vi "Log In 2.0.vi"(10 "required access level":i32, 11 "Program Root Path":path=path "C:/Labview Code") -> (0 "Password Out":string, 1 "User Name Out":string, 2 "Cancelled":bool, 3 "passed":bool, 4 "Level":i32)   [LabVIEW 2018]
panel:
  in  "User Name":string
  in  "Cancel":bool
  in  "Ok":bool
  in  "Password":string
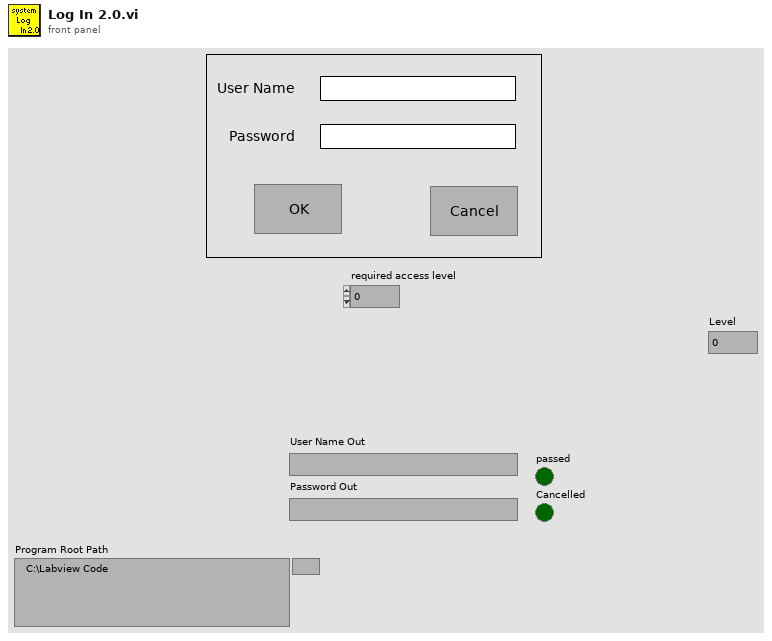
[diagram p1: front panel]
types:
  T1 = cluster{"Program Root Path":path, "Cancelled":bool, "Passed":bool, "User Names":string[], "Passwords":string[], "User Name Index":i32, "access levels":i32[]}
  T2 = typedef "eventvkey.ctl" = enum16{"ASCII", "Enter", "Return", "Shift", "Ctrl", "Alt", "Cmd", "Opt", "Caps", "NumLock", "Clear", "Break", "Up", "Down", "Left", "Right", "Insert", "Delete", "Home", "End", "PageUp", "PageDown", "Escape", "Help", "Pause", "ScrollLock", "F1", "F2", "F3", "F4", "F5", "F6", "F7", "F8", "F9", "F10", "F11", "F12", "F13", "F14", "F15", "F16", "F17", "F18", "F19", "F20", "F21", "F22", "F23", "F24", "Play", "VolumeUp", "VolumeDown", "Mute", "Two Byte Char"}
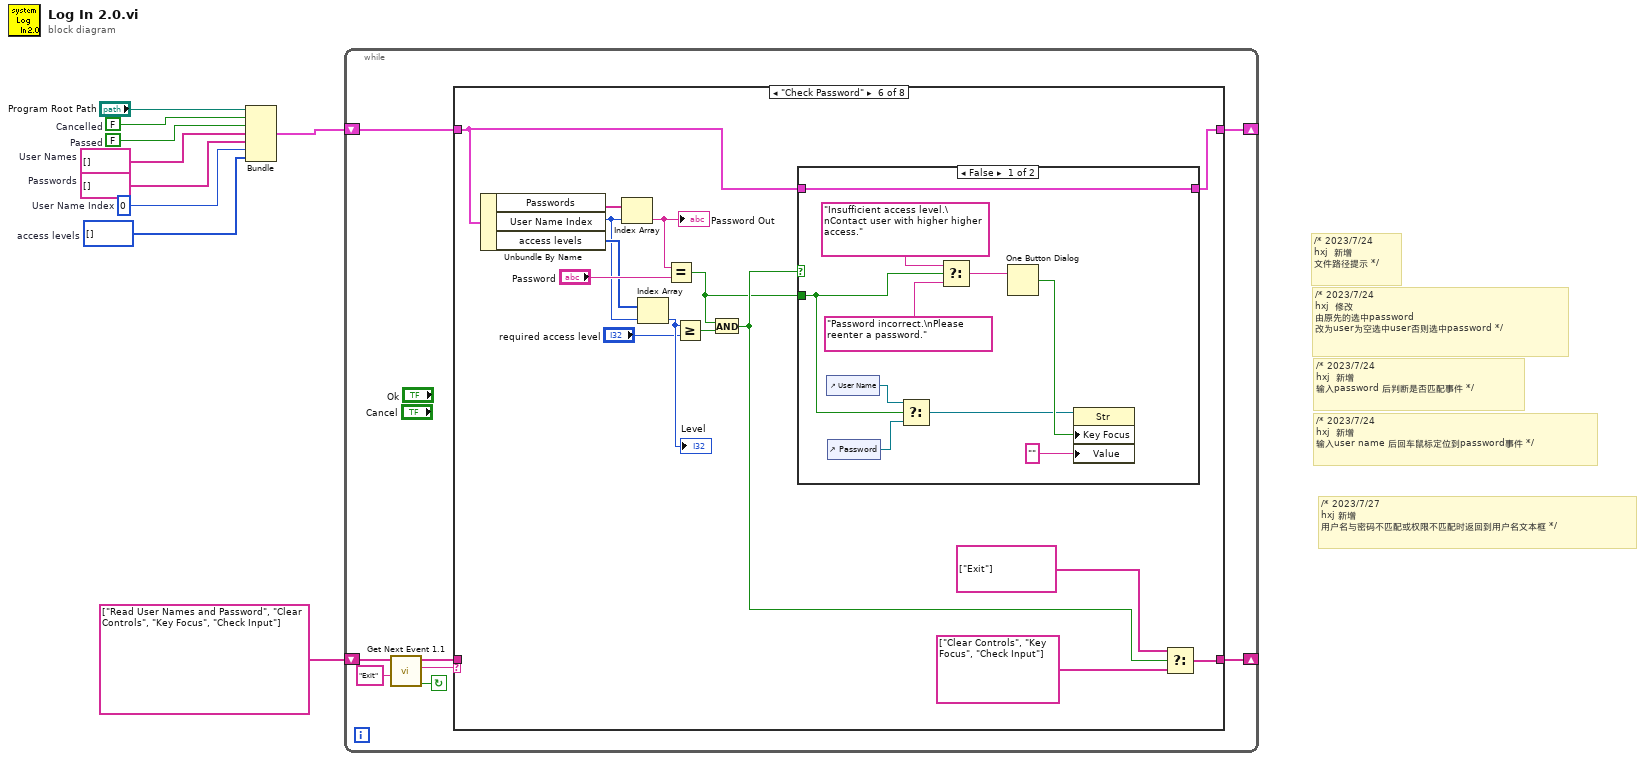
[diagram p0: block diagram]
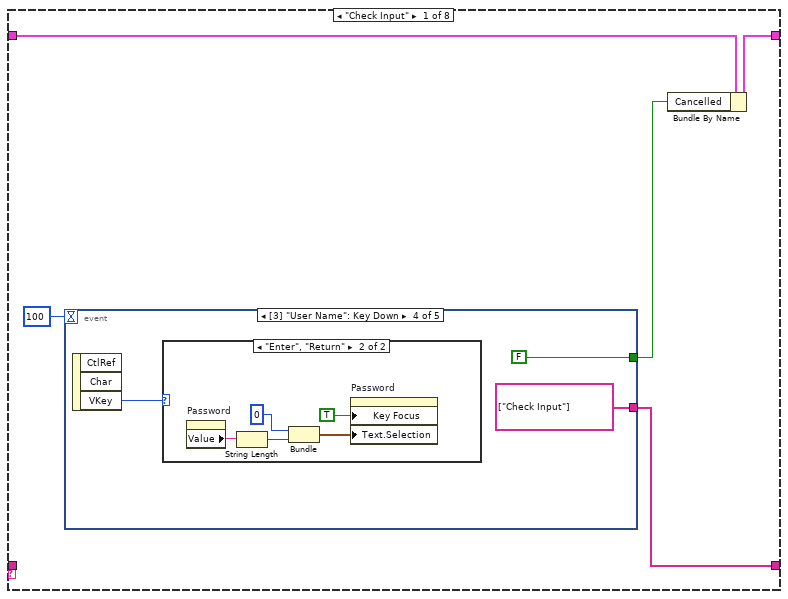
[diagram p2: hidden frame]
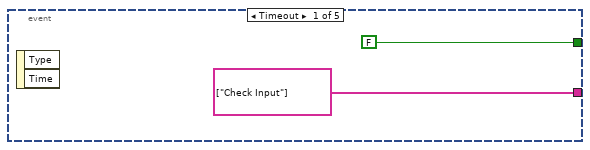
[diagram p3: hidden frame]
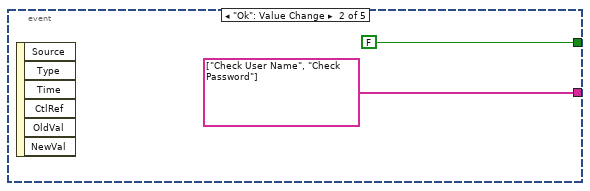
[diagram p4: hidden frame]
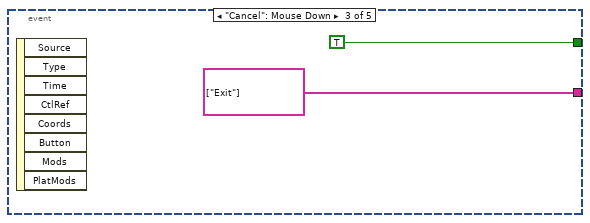
[diagram p5: hidden frame]
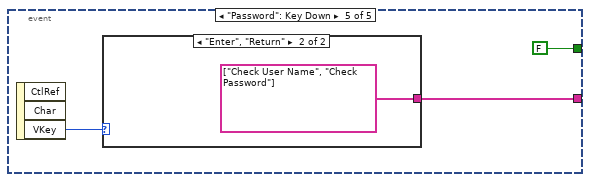
[diagram p7: hidden frame]
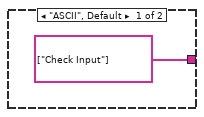
[diagram p8: hidden frame]
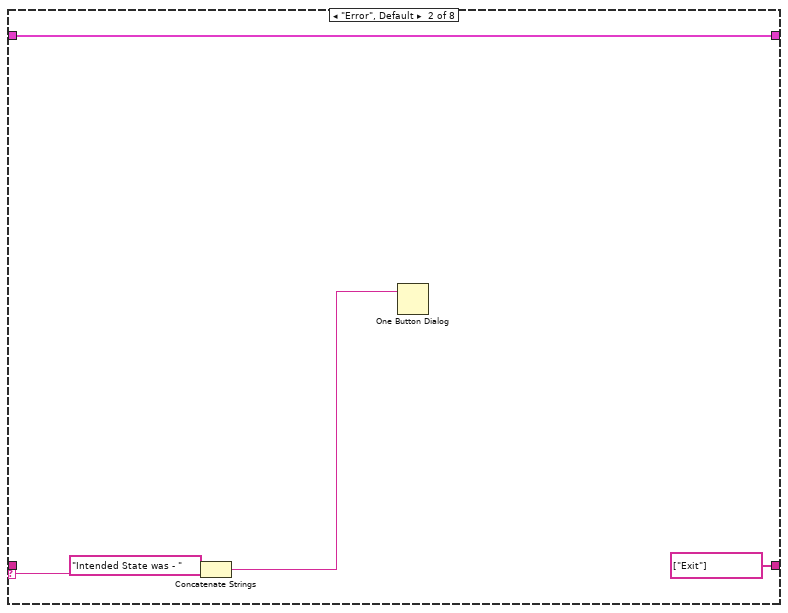
[diagram p9: hidden frame]
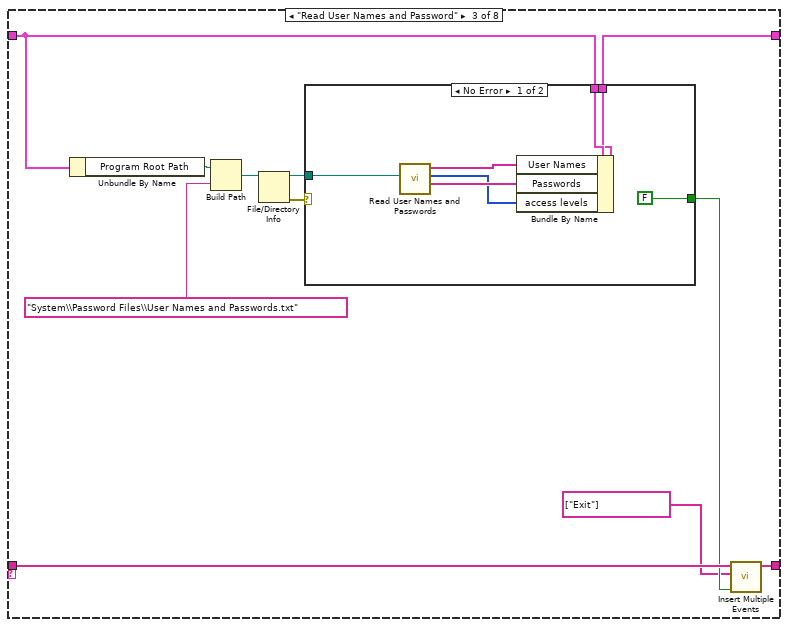
[diagram p10: hidden frame]
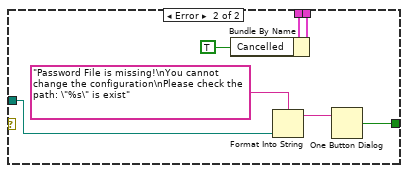
[diagram p11: hidden frame]
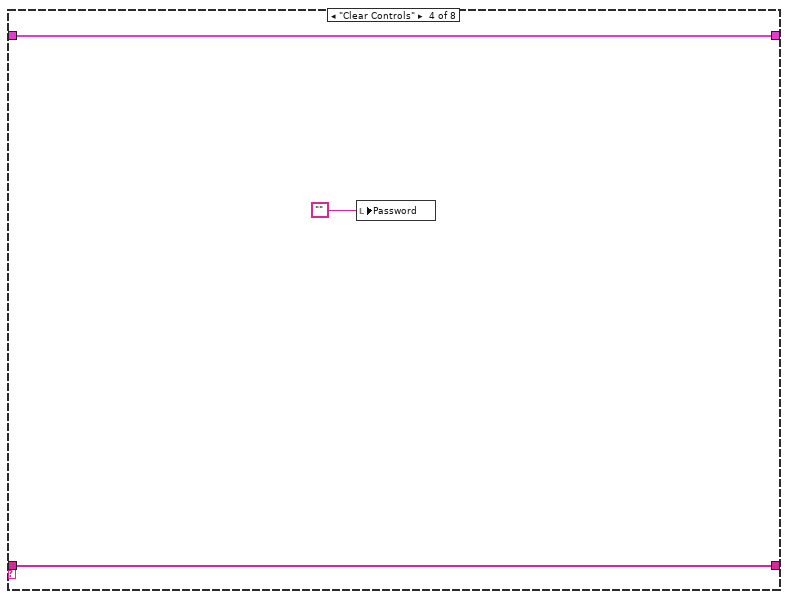
[diagram p12: hidden frame]
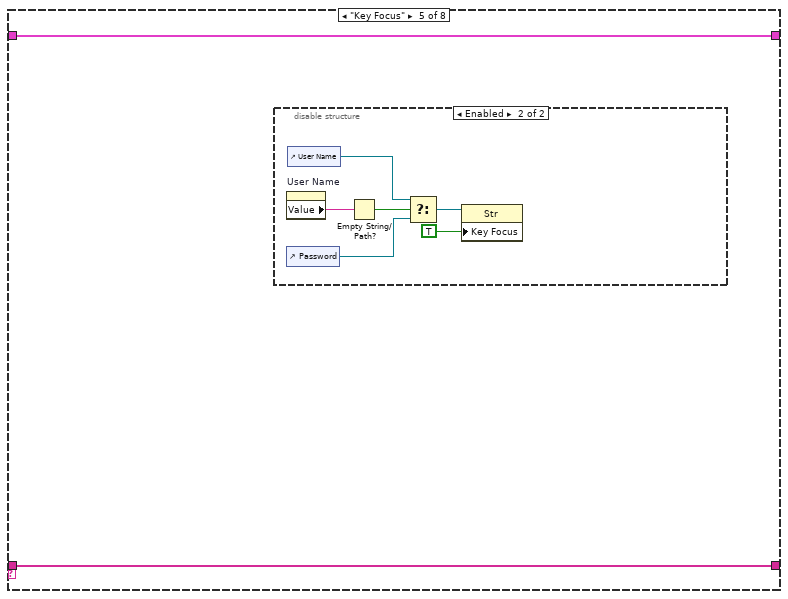
[diagram p13: hidden frame]
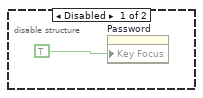
[diagram p14: hidden frame]
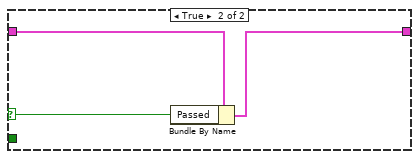
[diagram p15: hidden frame]
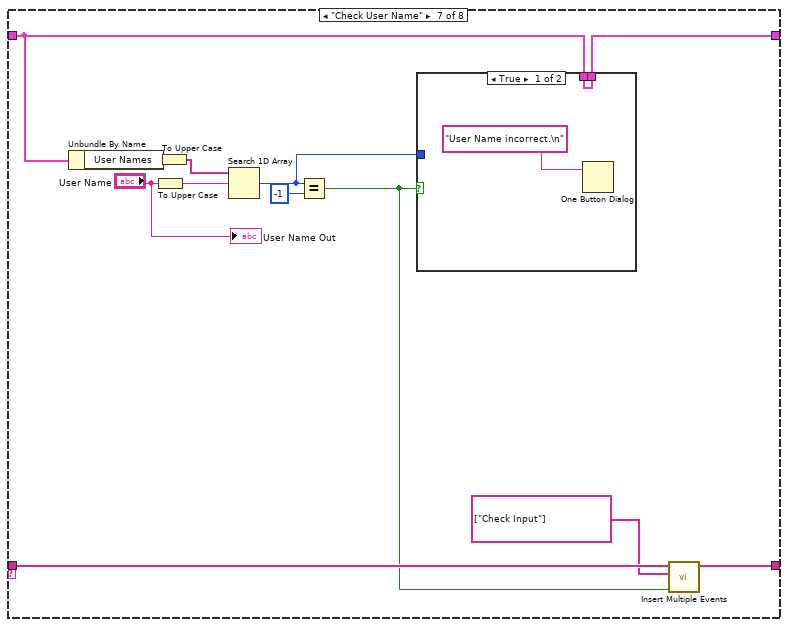
[diagram p16: hidden frame]
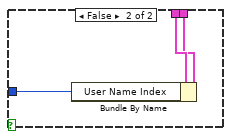
[diagram p17: hidden frame]
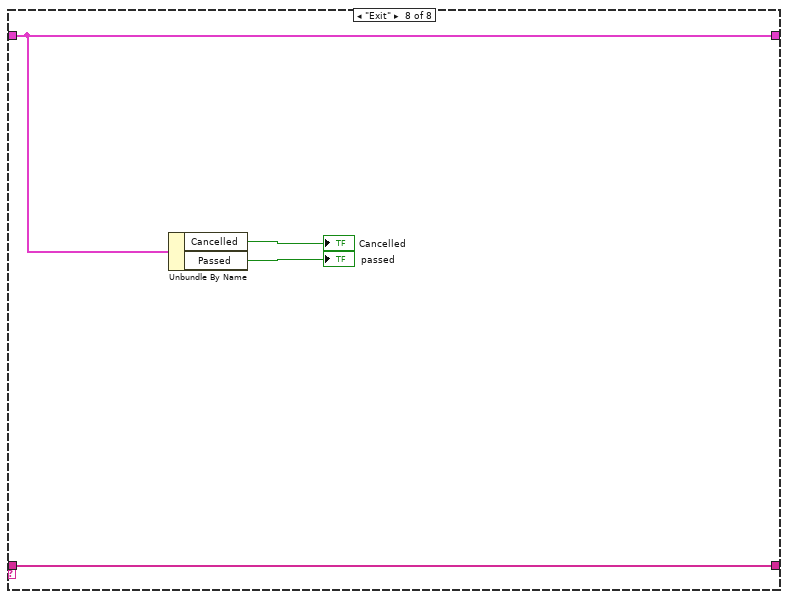
[diagram p18: hidden frame]
diagram:
  w1 = i32[] []  # access levels
  w2 = 0  # User Name Index
  w3 = string[] []  # User Names
  w4 = string[] []  # Passwords
  w5 = FALSE  # Passed
  w6 = FALSE  # Cancelled
  # "/* 2023/7/24\nhxj  修改\n由原先的选中password 改为user为空选中user否则选中password */"
  # "/* 2023/7/24\nhxj  新增\n文件路径提示 */"
  # "/* 2023/7/24\nhxj  新增\n输入user name 后回车鼠标定位到password事件 */"
  # "/* 2023/7/24\nhxj  新增\n输入password 后判断是否匹配事件 */"
  # "/* 2023/7/27\nhxj 新增\n用户名与密码不匹配或权限不匹配时返回到用户名文本框 */"
  n1 = Bundle("Program Root Path"="Program Root Path", "Cancelled"=w6, "Passed"=w5, "User Names"=w3, "Passwords"=w4, "User Name Index"=w2, "access levels"=w1) -> (w7:T1)  [unwired: 1 in]
  n2 = while {
    shift-right: [w11] -> _
    shift-left: w7 -> [w12]
    shift-right: [w13] -> _
    shift-left: string[] ["Read User Names and Password", "Clear Controls", "Key Focus", "Check Input"] ("event queue out") -> [w15]
    stop <- w17 continue-if-true
    n3 = call "Get Next Event 1.1.vi"("Exit Event"="Exit", "event queue in"=w15) -> ("Condition (Exit:F)"=w17:bool, "next event"=w16:string, "event queue out"=w14:string[])  [unwired: 6 in, 1 out]
    n4 = case shown="\"Check Password\"" w16 {
      selector: w16 -> [_ w44 _ _ _ _ _ _]
      tunnel: [w20 string[] ["Exit"] ("event queue out") w52 w73 w76 w95 w115 w132] -> w13
      tunnel: w14 -> [_ _ w51 w73 w76 _ w114 w132]
      tunnel: w12 -> [w22 w45 w56 w74 w75 w97 w122 w131]
      tunnel: [w21 w45 w55 w74 w75 w98 w123 w131] -> w11
      frame "Check Input" {
        n5 = event shown="[3] \"User Name\": Key Down" {
          selector: _ -> [_ _ _ _ _]
          dyn-events: _ -> [_ _ _ _ _]
          timeout: 100 -> [_ _ _ _ _]
          tunnel: [string[] ["Check Input"] ("Events to Insert") string[] ["Check User Name", "Check Password"] ("Events to Insert") string[] ["Exit"] ("Events to Insert") string[] ["Check Input"] ("Events to Insert") w38] -> w20
          tunnel: [FALSE FALSE TRUE FALSE FALSE] -> w18
          event Timeout {
            n6 = event-data() -> ()  [unwired: 1 in, 2 out]
          }
          event "Ok": Value Change {
            n7 = event-data() -> ()  [unwired: 1 in, 6 out]
          }
          event "Cancel": Mouse Down {
            n8 = event-data() -> ()  [unwired: 1 in, 8 out]
          }
          event "User Name": Key Down {
            n9 = event-data() -> ("VKey"=w31:T2)  [unwired: 1 in, 2 out]
            n10 = case shown="\"Enter\", \"Return\"" w31 {
              frame "ASCII", Default {
              }
              frame "Enter", "Return" {
                n11 = property on="Password" class="Str"() -> ("Value"=w36:string)  [unwired: 2 in, 2 out]
                n12 = String Length(string=w36) -> (length=w35:i32)
                n13 = Bundle(0, w35) -> (w33:cluster{i32, i32})  [unwired: 1 in]
                n14 = property on="Password" class="Str"("Key Focus"=TRUE ("键选中"), "Text.Selection"=w33) -> ()  [unwired: 2 in, 2 out]
              }
            }
          }
          event "Password": Key Down {
            n15 = event-data() -> ("VKey"=w39:T2)  [unwired: 1 in, 2 out]
            n16 = case shown="\"Enter\", \"Return\"" w39 {
              tunnel: [string[] ["Check Input"] ("Events to Insert") string[] ["Check User Name", "Check Password"] ("Events to Insert")] -> w38
              frame "ASCII", Default {
              }
              frame "Enter", "Return" {
              }
            }
          }
        }
        n17 = Bundle By Name(cluster=w22, "Cancelled"=w18) -> (w21:T1)
      }
      frame "Error", Default {
        n18 = Concatenate Strings("Intended State was - " ("string"), w44) -> (w43:string)
        n19 = One Button Dialog(message=w43) -> ()  [unwired: 1 in, 1 out]
      }
      frame "Read User Names and Password" {
        n20 = Unbundle By Name(w56) -> ("Program Root Path"=w48:path)
        n21 = Build Path(base path=w48, name or relative path="System\\Password Files\\User Names and Passwords.txt") -> (appended path=w47:path)
        n22 = File/Directory Info(path=w47) -> (path out=w53:path, error out=w54:errorcluster)  [unwired: 1 in, 5 out]
        n23 = case shown="No Error" w54 {
          tunnel: w56 -> [w64 w71]
          tunnel: [w63 w70] -> w55
          tunnel: w53 -> [w61 w67]
          tunnel: [FALSE ("true") w68] -> w50
          frame No Error {
            n24 = call "Read User Names and Passwords.vi"("Base Path"=w61) -> ("Passwords"=w59:string[], "access levels"=w58:i32[], "User Names"=w60:string[])  [unwired: 8 in]
            n25 = Bundle By Name(cluster=w64, "User Names"=w60, "Passwords"=w59, "access levels"=w58) -> (w63:T1)
          }
          frame Error {
            n26 = Bundle By Name(cluster=w71, "Cancelled"=TRUE) -> (w70:T1)
            n27 = Format Into String(format string="Password File is missing!\nYou cannot change the configuration\nPlease check the path: \"%s\" is exist" ("message"), w67) -> (resulting string=w66:string)  [unwired: 2 in, 1 out]
            n28 = One Button Dialog(message=w66) -> (true=w68:bool)  [unwired: 1 in]
          }
        }
        n29 = call "Insert Multiple Events.vi"("Insert all? (T)"=w50, "Events to Insert"=string[] ["Exit"], "Event queue in"=w51) -> ("Event queue out"=w52:string[])  [unwired: 4 in]
      }
      frame "Clear Controls" {
        n30 = local write "Password"("") -> ()
      }
      frame "Key Focus" {
        n31 = disable-structure shown="Enabled" {
          frame Disabled {
            n32 = property on="Password" class="Str"("Key Focus"=TRUE) -> ()  [unwired: 2 in, 2 out]
          }
          frame Enabled {
            n33 = property on="User Name" class="Str"() -> ("Value"=w80:string)  [unwired: 2 in, 2 out]
            n34 = control-ref of="Password"() -> (w83:refnum<vi>)
            n35 = control-ref of="User Name"() -> (w82:refnum<vi>)
            n36 = Empty String/Path?(string/path=w80) -> (empty?=w81:bool)
            n37 = Select(t=w82, s=w81, f=w83) -> (s? t:f=w79:refnum<vi>)
            n38 = property class="Str"(reference=w79, "Key Focus"=TRUE ("键选中")) -> ()  [unwired: 1 in, 2 out]
          }
        }
      }
      frame "Check Password" {
        n39 = Unbundle By Name(w97) -> ("Passwords"=w92:string[], "User Name Index"=w89:i32, "access levels"=w90:i32[])
        n40 = Index Array(array=w92, index=w89) -> (element=w91:string)
        "Password Out" <- w91
        n41 = Index Array(array=w90, index=w89) -> (element=w88:i32)
        "Level" <- w88
        n42 = Equal?(x=w91, y="Password") -> (x = y?=w84:bool)
        n43 = Greater Or Equal?(x=w88, y="required access level") -> (x >= y?=w86:bool)
        n44 = And(x=w84, y=w86) -> (x .and. y?=w85:bool)
        n45 = case shown="False" w85 {
          selector: w85 -> [_ w109]
          tunnel: w97 -> [w108 w111]
          tunnel: [w108 w110] -> w98
          tunnel: w84 -> [w104 _]
          frame False {
            n46 = control-ref of="User Name"() -> (w103:refnum<vi>)
            n47 = control-ref of="Password"() -> (w102:refnum<vi>)
            n48 = Select(t=w103, s=w104, f=w102) -> (s? t:f=w100:refnum<vi>)
            n49 = Select(t="Insufficient access level.\nContact user with higher higher access." ("message"), s=w104, f="Password incorrect.\nPlease reenter a password." ("message")) -> (s? t:f=w106:string)
            n50 = One Button Dialog(message=w106) -> (true=w101:bool)  [unwired: 1 in]
            n51 = property class="Str"(reference=w100, "Key Focus"=w101, "Value"="") -> ()  [unwired: 1 in, 2 out]
          }
          frame True {
            n52 = Bundle By Name(cluster=w111, "Passed"=w109) -> (w110:T1)
          }
        }
        n53 = Select(t=string[] ["Exit"] ("event queue out"), s=w85, f=string[] ["Clear Controls", "Key Focus", "Check Input"] ("event queue out")) -> (s? t:f=w95:string[])
      }
      frame "Check User Name" {
        n54 = Unbundle By Name(w122) -> ("User Names"=w121:string[])
        n55 = To Upper Case(1:"User Name") -> (0:w117:string)
        n56 = To Upper Case(1:w121) -> (0:w118:string[])
        n57 = Search 1D Array(1D array=w118, element=w117) -> (index of element=w119:i32)  [unwired: 1 in]
        n58 = Equal?(x=w119, y=-1) -> (x = y?=w113:bool)
        n59 = case shown="True" w113 {
          tunnel: w122 -> [w125 w128]
          tunnel: [w125 w127] -> w123
          tunnel: w119 -> [_ w126]
          frame True {
            n60 = One Button Dialog(message="User Name incorrect.\n") -> ()  [unwired: 1 in, 1 out]
          }
          frame False {
            n61 = Bundle By Name(cluster=w128, "User Name Index"=w126) -> (w127:T1)
          }
        }
        n62 = call "Insert Multiple Events.vi"("Insert all? (T)"=w113, "Events to Insert"=string[] ["Check Input"], "Event queue in"=w114) -> ("Event queue out"=w115:string[])  [unwired: 4 in]
        "User Name Out" <- "User Name"
      }
      frame "Exit" {
        n63 = Unbundle By Name(w131) -> ("Cancelled"=→"Cancelled":bool, "Passed"=→"passed":bool)
      }
    }
  }
